vi "MessageSender.vi"(0 "STOMP In":refnum<class "STOMP.lvclass">, 5 "error in (no error)":errorcluster) -> (14 "STOMP out":refnum<class "STOMP.lvclass">, 19 "error out":errorcluster)   [LabVIEW 2017, in "LabVIEW STOMP.lvlib" / "STOMP.lvclass"]
uses:
  STOMP.lvclass
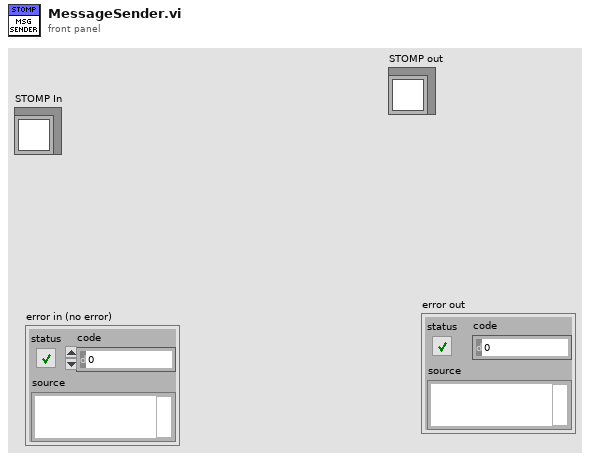
[diagram p1: front panel]
types:
  T1 = typedef "STOMP Connection Manager.lvclass/ObjectAttributes.ctl" = cluster{"address":string, "port":u16, "ConnectionRef":refnum<k5>, "messageQueue":refnum<queue>, "receiptQueue":refnum<queue>, "errorQueue":refnum<queue>, "sendQueue":refnum<queue>, "currentReceiptNumber":u64, "currentSubscriptionId":u64, "closeConnection":bool, "activeSubscriptions":T2[]}
  T2 = typedef "LabVIEW STOMP.lvlib/STOMP.lvclass/Type_ActiveSubscription.ctl" = cluster{"id":u64, "receipt":bool, "Destination":string, "ack":T3, "headers":T4[]}
  T3 = typedef "LabVIEW STOMP.lvlib/STOMP.lvclass/Type_AckHeader.ctl" = enum16{"auto", "client", "client-individual"}
  T4 = typedef "LabVIEW STOMP.lvlib/STOMP.lvclass/Type_FrameHeader.ctl" = cluster{"Header":string, "Value":string}
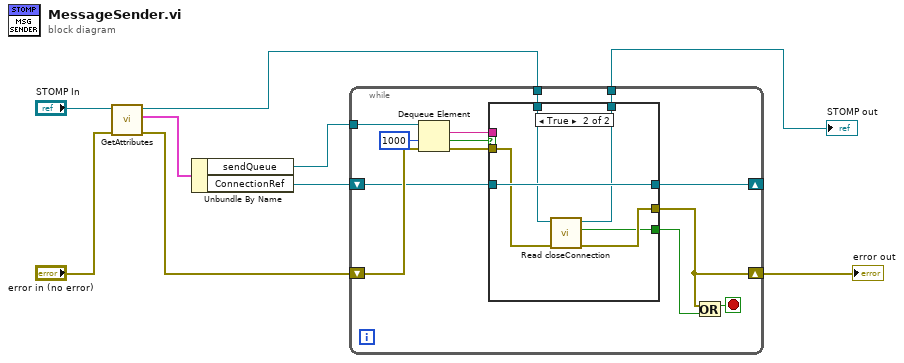
[diagram p0: block diagram]
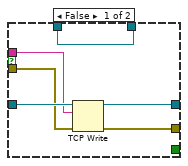
[diagram p2: hidden frame]
diagram:
  n1 = call-dynamic "GetAttributes.vi"("error in (no error)"="error in (no error)", "STOMP in"="STOMP In") -> ("error out"=w2:errorcluster, "attributes"=w4:T1, "STOMP out"=w1:refnum<class "STOMP.lvclass">)  [unwired: 7 in]
  n2 = Unbundle By Name(w4) -> ("sendQueue"=w8:refnum<queue>, "ConnectionRef"=w9:refnum<k5>)
  n3 = while {
    shift-right: [w17] -> _
    shift-left: w9 -> [w20]
    tunnel: w8 -> [w22]
    shift-right: [w18] -> w7
    shift-left: w2 -> [w21]
    tunnel: w1 -> [w13]
    tunnel: [w12] -> w6
    stop <- w11 stop-if-true
    n4 = Dequeue Element(queue=w22, timeout in ms (-1)=1000, error in (no error)=w21) -> (element=w19:string, timed out?=w14:bool, error out=w16:errorcluster)  [unwired: 1 out]
    n5 = case shown="True" w14 {
      tunnel: w20 -> [w28 w34]
      tunnel: w19 -> [w27 _]
      tunnel: [w26 w33] -> w18
      tunnel: [w25 w34] -> w17
      tunnel: w16 -> [w24 w32]
      tunnel: w13 -> [w23 w31]
      tunnel: [w23 w30] -> w12
      tunnel: [_ w29] -> w10
      frame False {
        n6 = TCP Write(connection ID=w28, data in=w27, error in (no error)=w24) -> (connection ID out=w25:refnum<k5>, error out=w26:errorcluster)  [unwired: 1 in, 1 out]
      }
      frame True {
        n7 = call-dynamic "Read closeConnection.vi"("error in (no error)"=w32, "STOMP in"=w31) -> ("error out"=w33:errorcluster, "closeConnection"=w29:bool, "STOMP out"=w30:refnum<class "STOMP.lvclass">)  [unwired: 7 in]
      }
    }
    n8 = Or(x=w18, y=w10) -> (x .or. y?=w11:bool)
  }
  "error out" <- w7
  "STOMP out" <- w6
